vi "New Image.vi"(4 "ImageTimestamp":timestamp, 6 "Camera Name":string, 8 "error in (no error)":errorcluster, 9 "Frame Nr":u32, 10 "Image":T1, 11 "HIJ Vision Camera App in":refnum<class "HIJ Vision Camera App.lvclass">) -> (0 "error out":errorcluster, 3 "HIJ Vision Camera App out":refnum<class "HIJ Vision Camera App.lvclass">)   [LabVIEW 2020, in "HIJ Vision Camera App.lvlib" / "HIJ Vision Camera App.lvclass"]
uses:
  HIJ Vision Camera App.lvclass
  C:/Users/AlexK/work/LabVIEW Programme/POLARIS CAM Log Abw und E/Submodules/HIJ Vision/Application Base Actors/HIJ Vision Application/HIJ Vision Application/HIJ Vision Application.lvclass
  <vilib>/vision/Image Controls.llb/IMAQ Image.ctl
  HIJ Vision Application/HIJ Vision Application/HIJ Vision Application.lvclass/HIJ Vision Application.ctl
  HIJ Vision Camera App.lvclass/HIJ Vision Camera App.ctl
  Camera Actors/Camera Actor/ICamera Messages/New Image Msg/New Image Msg.lvclass/New Image Msg.ctl
  <vilib>/ActorFramework/Message Enqueuer/Message Enqueuer.lvclass/Message Enqueuer.ctl
  HIJ Vision Application/HIJ Vision Application/Read Display Enq.vi
  Write Frame Nr.vi
  Write ImageTimeStamp.vi
  HIJ Vision Application/HIJ Vision Application/Write Raw Image.vi
  <vilib>/ActorFramework/Message Enqueuer/Enqueue.vi
  Camera Actors/Camera Actor/ICamera Messages/New Image Msg/New Image Msg.lvclass
  C:/Program Files (x86)/National Instruments/LabVIEW 2020/vi.lib/ActorFramework/Message/Message.lvclass
  <vilib>/ActorFramework/Message Priority Queue/Priority Enqueue.vi
  <vilib>/ActorFramework/Message Enqueuer/Message Enqueuer.lvclass
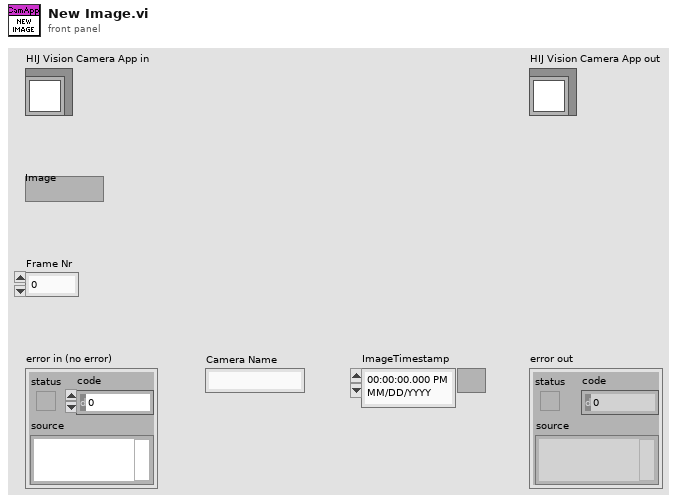
[diagram p1: front panel]
types:
  T1 = typedef "IMAQ Image.ctl" = refnum<image>
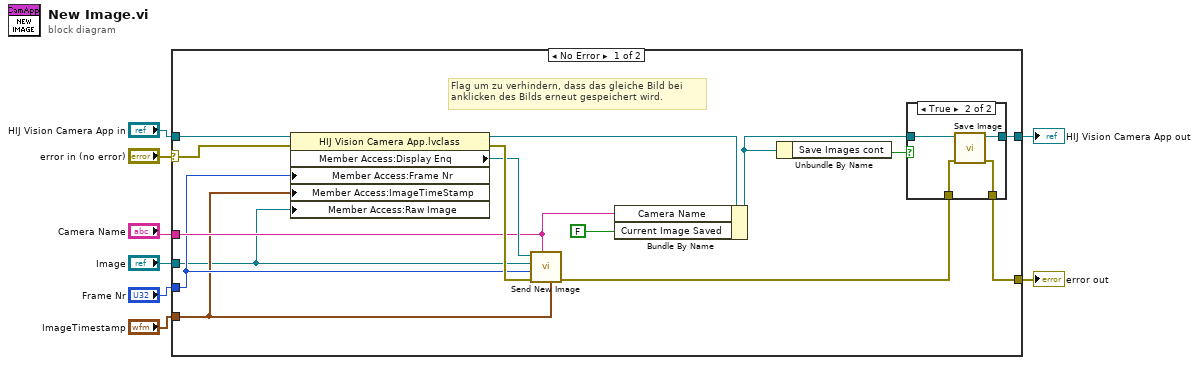
[diagram p0: block diagram]
diagram:
  n1 = case shown="No Error" "error in (no error)" {
    selector: "error in (no error)" -> [w19 w31]
    tunnel: [w10 w31] -> w7
    tunnel: [w12 w30] -> w5
    tunnel: "HIJ Vision Camera App in" -> [w22 w30]
    tunnel: "Image" -> [w14 _]
    tunnel: "Frame Nr" -> [w16 _]
    tunnel: "Camera Name" -> [w17 _]
    tunnel: "ImageTimestamp" -> [w15 _]
    frame No Error {
      # "Flag um zu verhindern, dass das gleiche Bild bei \nanklicken des Bilds erneut gespeichert wird."
      n2 = property class="HIJ Vision Camera App.lvclass"(reference=w22, error in=w19, "Member Access:Frame Nr"=w16, "Member Access:ImageTimeStamp"=w15, "Member Access:Raw Image"=w14) -> (reference out=w21:refnum<class "HIJ Vision Camera App.lvclass">, error out=w23:errorcluster, "Member Access:Display Enq"=w20:refnum<class "Message Enqueuer.lvclass">)
      n3 = call "Send New Image.vi"("ImageTimestamp"=w15, "Camera"=w17, "error in (no error)"=w23, "Buffer Number"=w16, "Image"=w14, "Message Enqueuer"=w20) -> ("error out"=w11:errorcluster)  [unwired: 4 in, 1 out]
      n4 = Bundle By Name(cluster=w21, "Camera Name"=w17, "Current Image Saved"=FALSE) -> (w13:refnum<class "HIJ Vision Camera App.lvclass">)
      n5 = Unbundle By Name(w13) -> ("Save Images cont"=w9:bool)
      n6 = case shown="True" w9 {
        tunnel: w13 -> [w25 w29]
        tunnel: [w25 w28] -> w12
        tunnel: w11 -> [w24 w27]
        tunnel: [w24 w26] -> w10
        frame False {
        }
        frame True {
          n7 = call-dynamic "Save Image.vi"("error in (no error)"=w27, "IMAQ Display in"=w29) -> ("error out"=w26:errorcluster, "IMAQ Display out"=w28:refnum<class "HIJ Vision Camera App.lvclass">)  [unwired: 8 in]
        }
      }
    }
    frame Error {
    }
  }
  "error out" <- w7
  "HIJ Vision Camera App out" <- w5
